vi "Config Units.vi"(8 "error in":errorcluster, 10 "Units (nS)":i32(ring)=1 items=["nanosiemens"=1, "dissipation factor"=2, "kilohms"=3, "gigohms"=4, "loss vector (jpF)"=5], 11 "VISA resource name":refnum<visa-resource-name>) -> (0 "error out":errorcluster, 3 "VISA resource name out":refnum<visa-resource-name>)   [LabVIEW 2018, in "Andeen-Hagerling 2700.lvlib"]
doc: "This VI selects the units that will be used to report the loss component of the measurements. Note that after setting units, the bridge will send the last measurement results in the new units."
uses:
  Andeen-Hagerling 2700.lvlib
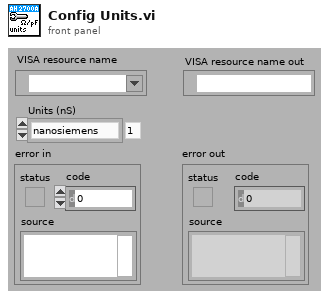
[diagram p1: front panel]
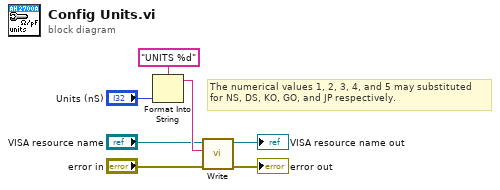
[diagram p0: block diagram]
diagram:
  # "The numerical values 1, 2, 3, 4, and 5 may substituted\nfor NS, DS, KO, GO, and JP respectively."
  n1 = Format Into String(format string="UNITS %d", "Units (nS)") -> (resulting string=w5:string)  [unwired: 2 in, 1 out]
  n2 = call "Write.vi"("error in"="error in", "command"=w5, "VISA resource name"="VISA resource name") -> ("error out"=→"error out":errorcluster, "VISA resource name out"=→"VISA resource name out":refnum<visa-resource-name>)  [unwired: 7 in]
